vi "solar_voy Unpack.vi"(0 "Voyager Refnum in":T7, 1 "CMD":enum8{"CMD", "TLM"}(ring), 5 "TCP Data":string, 7 "ID":u16, 11 "error in (no error)":errorcluster) -> (2 "HDR":T1, 3 "PACKET":T5 {"last_time" format="%<%H:%M:%S%3u %m/%d/%y>T"}, 4 "Voyager Refnum out":T7, 6 "Item Values":variant[](array[variant]), 8 "Item Values (LV Flattened Value)":string[](array[string]), 10 "Packet Index":i32, 15 "error out":errorcluster)   [LabVIEW 2018]
doc: "This unpacks the TCP Data into the registered packet. The Last Value items are updated including the timestamp and update count."
uses:
  solar_voy_ctl Voyager Refnum.ctl
  solar_voy_def/solar_voy_def_ctl ITEM TYPE.ctl
  type/solar_type Item Type.ctl
  solar_voy_def/solar_voy_def_ctl ITEM.ctl
  solar_voy_def/solar_voy_def_ctl PACKET_ID.ctl
  solar_voy_def/solar_voy_def_ctl PACKET.ctl
  solar_voy_def/solar_voy_def_ctl HDR.ctl
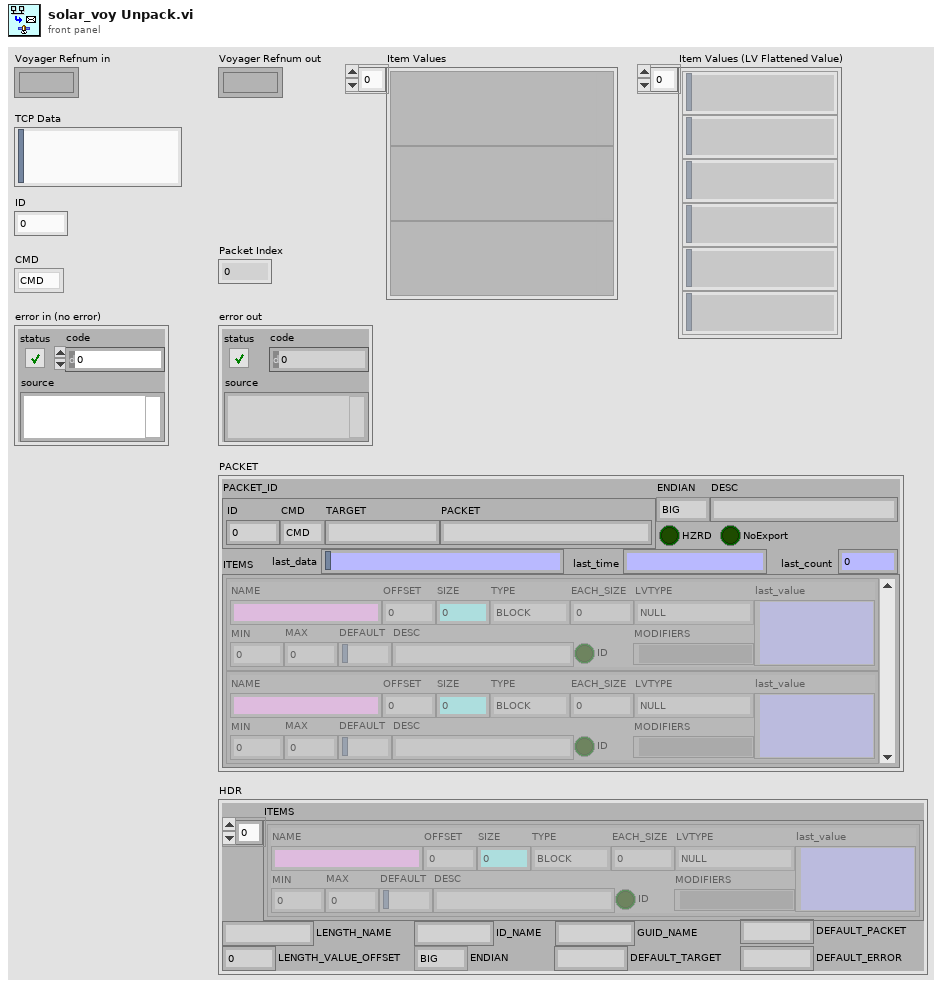
[diagram p1: front panel]
types:
  T1 = typedef "solar_voy_def_ctl HDR.ctl" = cluster{"ITEMS":T2[], "LENGTH_NAME":string, "LENGTH_VALUE_OFFSET":i32, "ID_NAME":string, "ENDIAN":enum8{"BIG", "LITTLE"}, "GUID_NAME":string, "DEFAULT_TARGET":string, "DEFAULT_PACKET":string, "DEFAULT_ERROR":string}
  T2 = typedef "solar_voy_def_ctl ITEM.ctl" = cluster{"NAME":string, "OFFSET":i32, "SIZE":i32, "TYPE":T3, "EACH_SIZE":i32, "LVTYPE":T4, "MIN":dbl, "MAX":dbl, "DEFAULT":string, "DESC":string, "ID":bool, "MODIFIERS":variant, "last_value":variant}
  T3 = typedef "solar_voy_def_ctl ITEM TYPE.ctl" = enum8{"BLOCK", "INT", "UINT", "FLOAT", "STRING"}
  T4 = typedef "solar_type Item Type.ctl" = enum16{"NULL", "UNKNOWN", "CLUSTER", "I8", "I16", "I32", "I64", "U8", "U16", "U32", "U64", "U8_ENUM", "U16_ENUM", "U32_ENUM", "SGL", "DBL", "BOOLEAN", "STRING", "PATH", "VISA", "TAG", "TIME", "I8_1D", "I16_1D", "I32_1D", "I64_1D", "U8_1D", "U16_1D", "U32_1D", "U64_1D", "U8_ENUM_1D", "U16_ENUM_1D", "U32_ENUM_1D", "SGL_1D", "DBL_1D", "BOOLEAN_1D", "STRING_1D", "PATH_1D", "VISA_1D", "TAG_1D", "TIME_1D", "I8_2D", "I16_2D", "I32_2D", "I64_2D", "U8_2D", "U16_2D", "U32_2D", "U64_2D", "U8_ENUM_2D", "U16_ENUM_2D", "U32_ENUM_2D", "SGL_2D", "DBL_2D", "BOOLEAN_2D", "STRING_2D", "PATH_2D", "VISA_2D", "TAG_2D", "TIME_2D"}
  T5 = typedef "solar_voy_def_ctl PACKET.ctl" = cluster{"PACKET_ID":T6, "ENDIAN":enum8{"BIG", "LITTLE"}, "DESC":string, "HZRD":bool, "ITEMS":T2[], "NoExport":bool, "last_time":timestamp, "last_count":u32, "last_data":string}
  T6 = typedef "solar_voy_def_ctl PACKET_ID.ctl" = cluster{"ID":u16, "CMD":enum8{"CMD", "TLM"}, "TARGET":string, "PACKET":string}
  T7 = typedef "solar_voy_ctl Voyager Refnum.ctl" = refnum<k1>
  T8 = typedef "solar_voy_ctl Voyager.ctl" = cluster{"PACKETS":T5[], "COSMOS_Root":path, "CMD_HDR":T1, "TLM_HDR":T1, "TCPs":T9[], "VoyagerIDOffset":cluster{"VoyagerIDOffset":u16[], "Target Names":string[]}}
  T9 = typedef "solar_voy_ctl TCP.ctl" = cluster{"Connected":bool, "Port":u16, "Listener":refnum<k5>, "ServerIP":string, "TCP":refnum<k5>, "Setup":T10, "VIRefnum":refnum<vi>, "TARGETS_CMD":string[], "TARGETS_TLM":string[]}
  T10 = typedef "solar_voy_ctl Port Setup.ctl" = enum8{"SERVER", "CLIENT", "SERVER_CMD", "SERVER_TLM"}
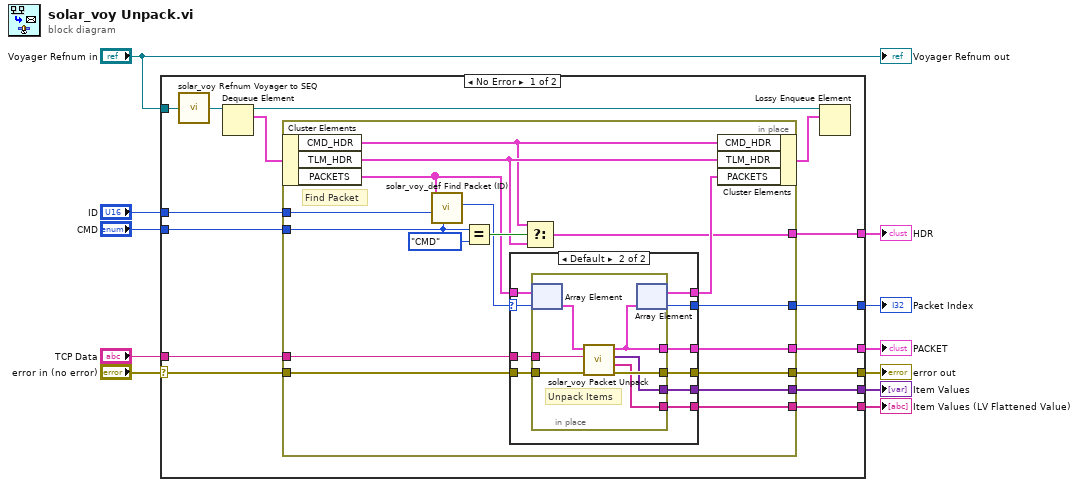
[diagram p0: block diagram]
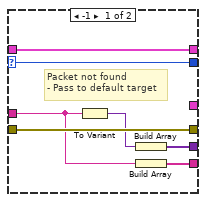
[diagram p2: hidden frame]
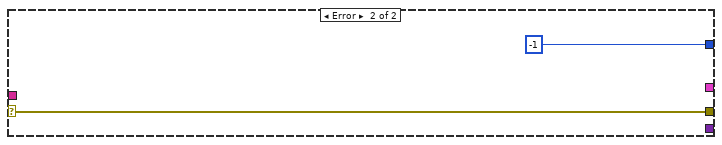
[diagram p3: hidden frame]
diagram:
  n1 = case shown="No Error" "error in (no error)" {
    selector: "error in (no error)" -> [w21 w69]
    tunnel: [w26 -1 ("Index")] -> w11
    tunnel: [w25 w69] -> w10
    tunnel: "CMD" -> [w24 _]
    tunnel: "ID" -> [w23 _]
    tunnel: "TCP Data" -> [w22 _]
    tunnel: "Voyager Refnum in" -> [w19 _]
    tunnel: [w15 _] -> w4
    tunnel: [w14 _] -> w3
    tunnel: [w13 _] -> w2
    tunnel: [w12 _] -> w1
    frame No Error {
      n2 = call "solar_voy Refnum Voyager to SEQ.vi"("Voyager Refnum"=w19) -> ("Voyager SEQ"=w16:refnum<queue>)
      n3 = Dequeue Element(queue=w16) -> (queue out=w17:refnum<queue>, element=w18:T8)  [unwired: 2 in, 2 out]
      n4 = in-place {
        in-place-border: w21 -> [w43]
        in-place-border: [w42] -> w25
        in-place-border: w23 -> [w41]
        in-place-border: w24 -> [w38]
        in-place-border: w22 -> [w36]
        in-place-border: [w33] -> w26
        in-place-border: [w32] -> w15
        in-place-border: [w29] -> w14
        in-place-border: [w28] -> w13
        in-place-border: [w27] -> w12
        # "Find Packet"
        n5 = in-place-cluster #1(w18) -> ("CMD_HDR"=w30:T1, "TLM_HDR"=w31:T1, "PACKETS"=w34:T5[])
        n6 = call "solar_voy_def Find Packet (ID).vi"("CMD"=w38, "ID"=w41, "PACKETS"=w34) -> ("Index"=w37:i32)  [unwired: 8 in]
        n7 = Equal?(x=w38, y=enum8{"CMD", "TLM"}."CMD") -> (x = y?=w39:bool)
        n8 = case shown="Default" w37 {
          selector: w37 -> [w48 w58]
          tunnel: w43 -> [w50 w60]
          tunnel: [w50 w59] -> w42
          tunnel: w36 -> [w45 w57]
          tunnel: w34 -> [w49 w56]
          tunnel: [w49 w55] -> w35
          tunnel: [w48 w54] -> w33
          tunnel: [_ w53] -> w32
          tunnel: [w44 w52] -> w28
          tunnel: [w46 w51] -> w27
          frame -1 {
            # "Packet not found\n- Pass to default target"
            n9 = To Variant(anything=w45) -> (Variant=w47:variant)
            n10 = Build Array(w47) -> (w46:variant[])
            n11 = Build Array(w45) -> (w44:string[])
          }
          frame Default {
            n12 = in-place {
              in-place-border: w60 -> [w67]
              in-place-border: [w66] -> w59
              in-place-border: w57 -> [w64]
              in-place-border: [w63] -> w53
              in-place-border: [w62] -> w52
              in-place-border: [w61] -> w51
              # "Unpack Items"
              n13 = in-place-array #2(w56, w58) -> (w65:T5)
              n14 = call "solar_voy Packet Unpack.vi"("error in (no error)"=w67, "TCP Message Read"=w64, "PACKET in"=w65) -> ("error out"=w66:errorcluster, "Item Values (TCP)"=w62:string[], "Item Values"=w61:variant[], "PACKET out"=w63:T5)  [unwired: 5 in]
              n15 = in-place-array #2(w63) -> (w55:T5[], w54:i32)
            }
          }
        }
        n16 = Select(t=w30, s=w39, f=w31) -> (s? t:f=w29:T1)
        n17 = in-place-cluster #1("CMD_HDR"=w30, "TLM_HDR"=w31, "PACKETS"=w35) -> (w20:T8)
      }
      n18 = Lossy Enqueue Element(queue=w17, element=w20) -> ()  [unwired: 1 in, 4 out]
    }
    frame Error {
    }
  }
  "Packet Index" <- w11
  "error out" <- w10
  "PACKET" <- w4
  "HDR" <- w3
  "Item Values (LV Flattened Value)" <- w2
  "Item Values" <- w1
  "Voyager Refnum out" <- "Voyager Refnum in"
